vi "Write Gas.vi"(8 "error in":errorcluster, 10 "Gas":T1, 11 "Alicat in":refnum<class "Alicat.lvclass">) -> (0 "error out":errorcluster, 3 "Alicat out":refnum<class "Alicat.lvclass">)   [LabVIEW 2015, in "Alicat.lvlib" / "Alicat.lvclass"]
uses:
  Alicat.lvclass
  Controls/Gas.ctl
  Alicat.lvclass/Alicat.ctl
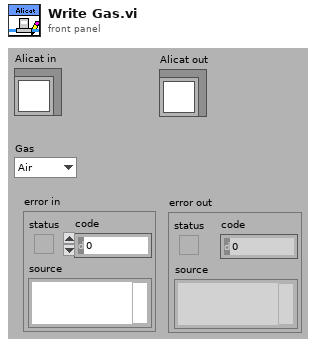
[diagram p1: front panel]
types:
  T1 = typedef "Alicat.lvlib/Alicat.lvclass/Gas.ctl" = enum16{"Air", "Ar", "CH4", "CO", "CO2", "C2H6", "H2", "He", "N2", "NO", "Ne", "O2", "C3H8", "n-C4H10", "C2H2", "C2H4", "i-C2H10", "Kr", "Xe"}
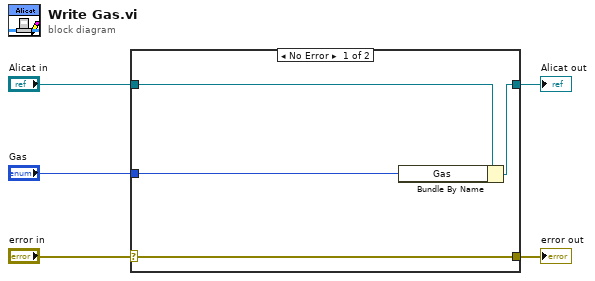
[diagram p0: block diagram]
diagram:
  n1 = case shown="No Error" "error in" {
    selector: "error in" -> [w9 w10]
    tunnel: [w9 w10] -> w4
    tunnel: [w7 w11] -> w2
    tunnel: "Alicat in" -> [w8 w11]
    tunnel: "Gas" -> [w6 _]
    frame No Error {
      n2 = Bundle By Name(cluster=w8, "Gas"=w6) -> (w7:refnum<class "Alicat.lvclass">)
    }
    frame Error {
    }
  }
  "error out" <- w4
  "Alicat out" <- w2
